vi "Trigger2Photon.vi"(11 "Refnum in":refnum<k21>) -> (0 "error out":errorcluster, 3 "Refnum out":refnum<k21>)   [LabVIEW 2013]
uses:
  <vilib>/DAQmx/write.llb/DAQmx Write (Digital Bool 1Line 1Point).vi
  <vilib>/DAQmx/miscellaneous.llb/DAQmx Fill In Error Info.vi
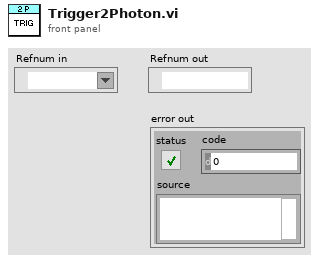
[diagram p1: front panel]
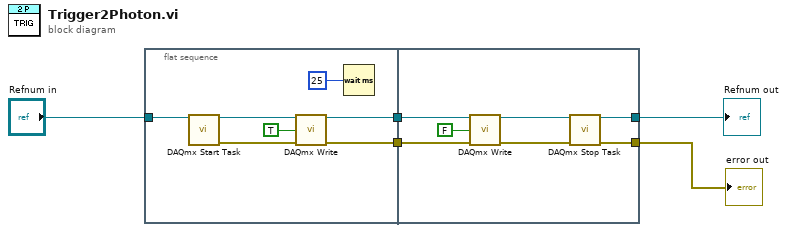
[diagram p0: block diagram]
diagram:
  n1 = flat-sequence {
    tunnel: [w10] -> w5
    tunnel: "Refnum in" -> [w8]
    tunnel: [w6] -> w2
    tunnel: w5 -> [w19]
    tunnel: [w16] -> w4
    tunnel: w2 -> [w15]
    tunnel: [w13] -> w1
    frame #0 {
      n2 = call <vilib>:"DAQmx Start Task.vi"("task/channels in"=w8) -> ("task out"=w9:refnum<k21>, "error out"=w7:errorcluster)  [unwired: 13 in]
      n3 = call-poly <vilib>:"DAQmx Write.vi"("task/channels in"=w9, "data"=TRUE, "error in"=w7) -> ("task out"=w10:refnum<k21>, "error out"=w6:errorcluster)  [unwired: 10 in, 1 out]
      n4 = Wait (ms)(milliseconds to wait=u32 25) -> ()  [unwired: 1 out]
    }
    frame #1 {
      n5 = call-poly <vilib>:"DAQmx Write.vi"("task/channels in"=w19, "data"=FALSE, "error in"=w15) -> ("task out"=w17:refnum<k21>, "error out"=w14:errorcluster)  [unwired: 10 in, 1 out]
      n6 = call <vilib>:"DAQmx Stop Task.vi"("task/channels in"=w17, "error in"=w14) -> ("task out"=w16:refnum<k21>, "error out"=w13:errorcluster)  [unwired: 12 in]
    }
  }
  "Refnum out" <- w4
  "error out" <- w1
